vi "LC-MISDK_UserCalibration_sub.vi"(5 ".NET refnum入力":refnum<k24>, 6 "Color Space":T9(ring), 7 "Clust refnum":refnum<vi>) -> ()   [LabVIEW 2015]
uses:
  C:/Users/e09031/Documents/GMA/LC-160/Labview/Sample_LC-MISDK/LC-MISDK.dll
  LC-MISDK.dll
panel:
  in  "After_B":T1
  in  "After_G":T2
  in  "After_R":T3
  in  "After_W":T4
  in  "Before_B":T5
  in  "Before_G":T6
  in  "Before_R":T7
  in  "Before_W":T8
  out "Error Message":string
  in  "EXIT":bool
  in  "Calib":bool
  in  "ID":string
  out "Calib.Ch":T10(ring)
  out "Type of Calibration":enum32{"Single-Point", "RGB", "WRGB"}(radio)
  # "Value before Calibration"
  # "Value after Calibration"
  # "Lavel1"
  # "Lavel2"
  # "Lavel3"
  # "Lavel1"
  # "Lavel2"
  # "Lavel3"
  # "White"
  # "White"
  # "Red"
  # "Red"
  # "Green"
  # "Green"
  # "Blue"
  # "Blue"
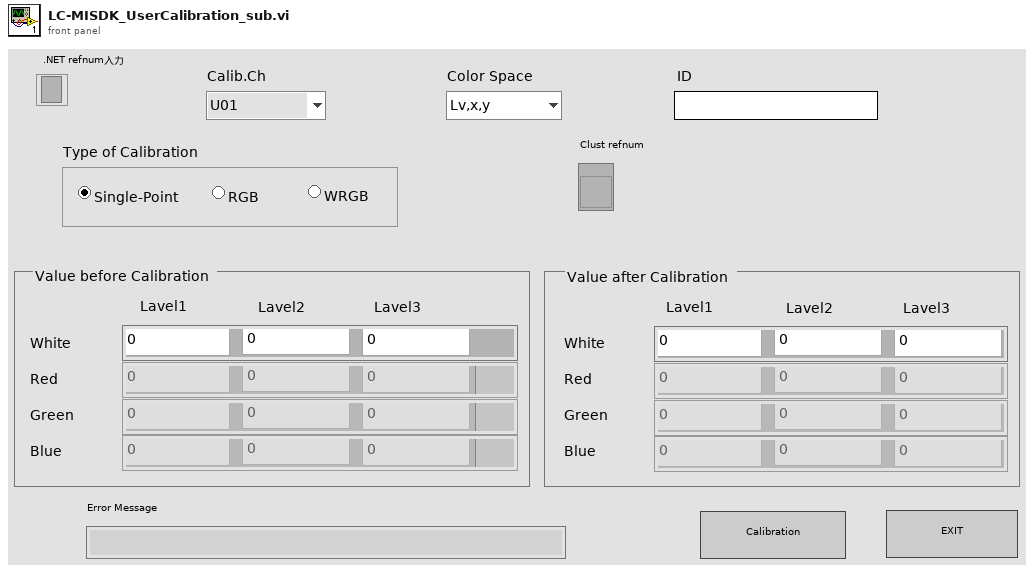
[diagram p1: front panel]
types:
  T1 = cluster{"After_B1":dbl, "After_B2":dbl, "After_B3":dbl}
  T2 = cluster{"After_G1":dbl, "After_G2":dbl, "After_G3":dbl}
  T3 = cluster{"After_R1":dbl, "After_R2":dbl, "After_R3":dbl}
  T4 = cluster{"After_W1":dbl, "After_W2":dbl, "After_W3":dbl}
  T5 = cluster{"before_B1":dbl, "Before_B":bool, "Before_B2":dbl, "Before_B3":dbl}
  T6 = cluster{"before_G1":dbl, "Before_G":bool, "Before_G2":dbl, "Before_G3":dbl}
  T7 = cluster{"before_R1":dbl, "Before_R":bool, "Before_R2":dbl, "Before_R3":dbl}
  T8 = cluster{"before_W1":dbl, "Before_W2":dbl, "Before_W3":dbl}
  T9 = enum16{"Lv,x,y", "Lv,u',v'", "Lv,Tcp,duv", "X,Y,Z", "Lv,λd,Pe"}
  T10 = enum16{"U01", "U02", "U03", "U04", "U05", "U06", "U07", "U08", "U09", "U10"}
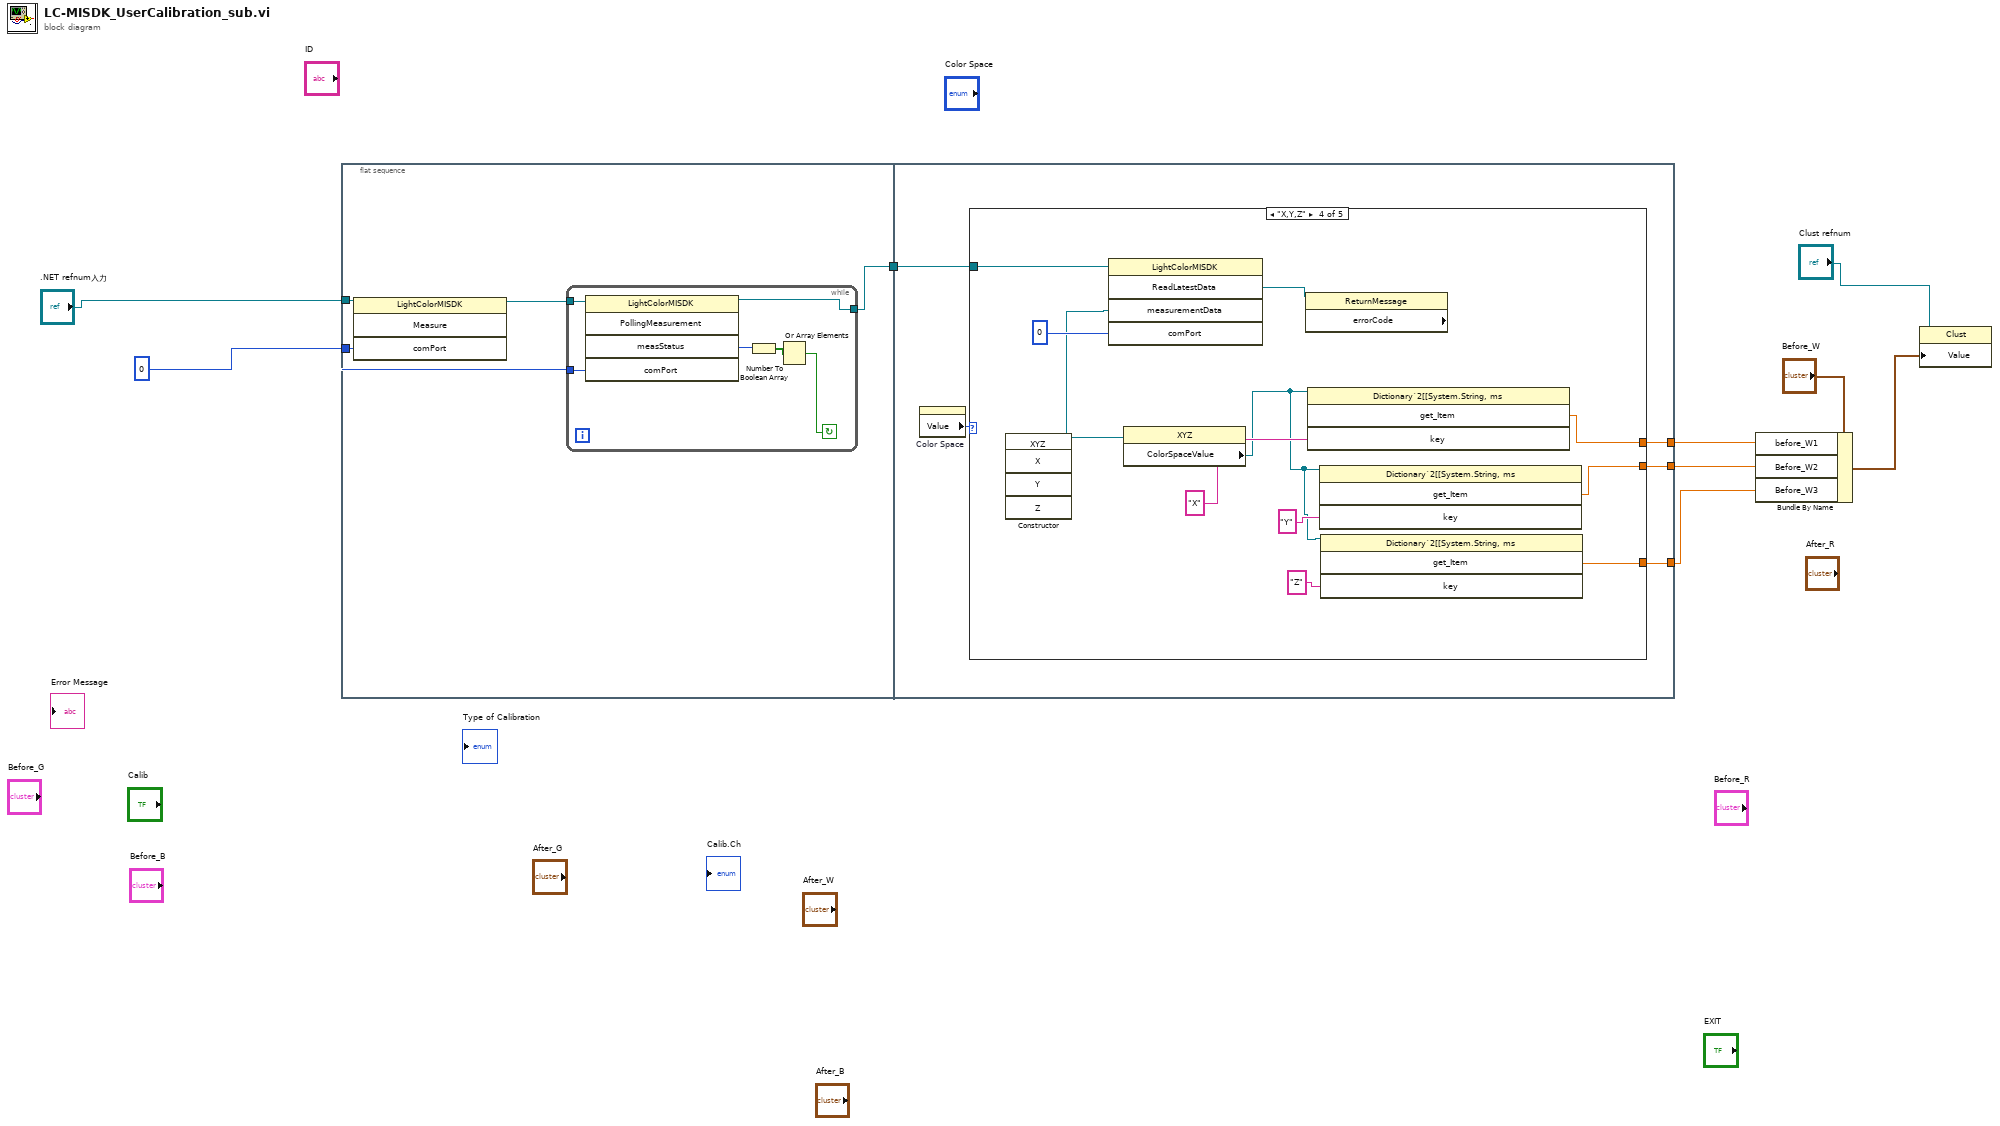
[diagram p0: block diagram]
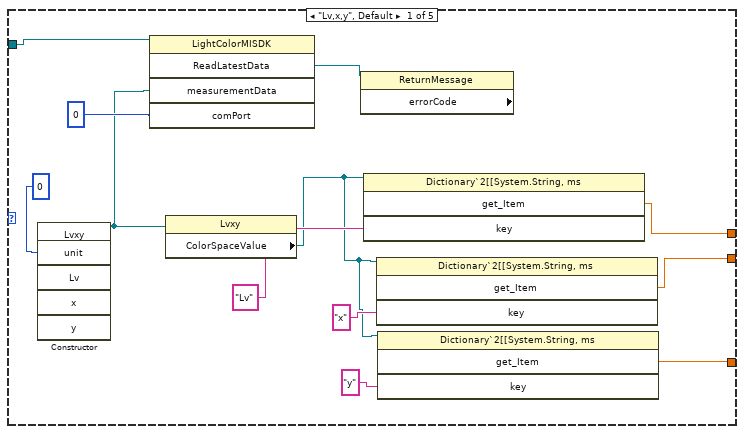
[diagram p2: hidden frame]
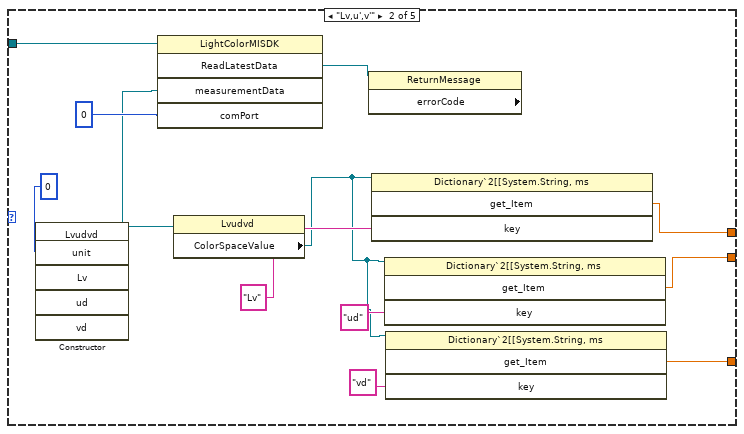
[diagram p3: hidden frame]
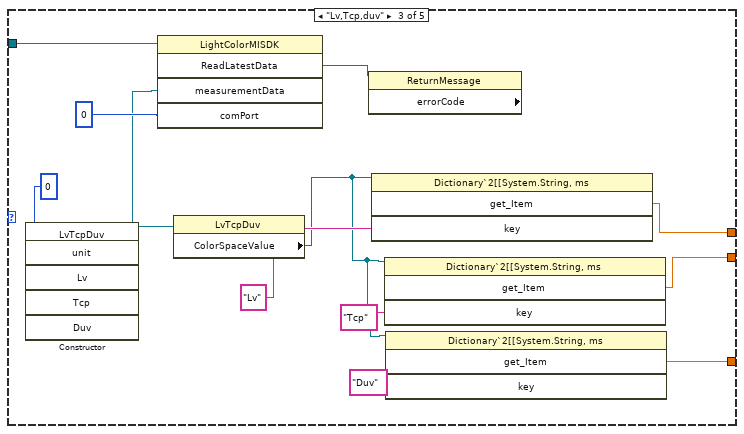
[diagram p4: hidden frame]
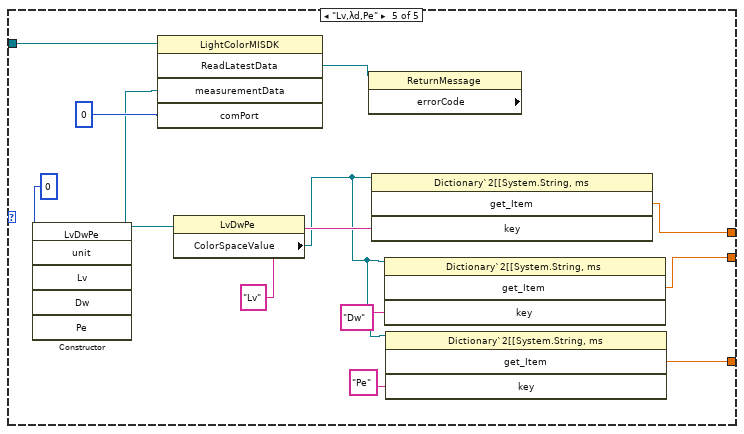
[diagram p5: hidden frame]
diagram:
  n1 = flat-sequence {
    tunnel: ".NET refnum入力" -> [w12]
    tunnel: 0 -> [w11]
    tunnel: [w10] -> w9
    tunnel: w9 -> [w24]
    tunnel: [w23] -> w8
    tunnel: [w22] -> w7
    tunnel: [w21] -> w6
    frame #0 {
      n2 = invoke on="インボークノード" class="LightColorMISDK" method="Measure"(reference=w12, "comPort"=w11) -> (reference out=w13:refnum<k24>)  [unwired: 2 in, 3 out]
      n3 = while {
        tunnel: [w18] -> w10
        tunnel: w13 -> [w17]
        tunnel: w11 -> [w14]
        stop <- w15 continue-if-true
        n4 = invoke on="インボークノード" class="LightColorMISDK" method="PollingMeasurement"(reference=w17, "comPort"=w14) -> (reference out=w18:refnum<k24>, "measStatus"=w19:i32)  [unwired: 3 in, 3 out]
        n5 = Number To Boolean Array(number=w19) -> (Boolean array=w16:bool[])
        n6 = Or Array Elements(Boolean array=w16) -> (logical OR=w15:bool)
      }
    }
    frame #1 {
      n7 = property on="Color Space" class="Enum （指定）"() -> ("Value"=w20:T9)  [unwired: 2 in, 2 out]
      n8 = case shown="\"X,Y,Z\"" w20 {
        tunnel: w24 -> [w28 w40 w52 w64 w75]
        tunnel: [w27 w39 w51 w63 w74] -> w23
        tunnel: [w26 w38 w50 w62 w73] -> w22
        tunnel: [w25 w37 w49 w61 w72] -> w21
        frame "Lv,x,y", Default {
          n9 = constructor class="Lvxy"("unit"=0) -> (reference out=w34:refnum<k24>)  [unwired: 6 in, 6 out]
          n10 = invoke on="インボークノード" class="LightColorMISDK" method="ReadLatestData"(reference=w28, "measurementData"=w34, "comPort"=0) -> ("ReadLatestData"=w35:refnum<k24>)  [unwired: 2 in, 4 out]
          n11 = property class="Lvxy"(reference=w34) -> ("ColorSpaceValue"=w31:refnum<k24>)  [unwired: 1 in, 2 out]
          n12 = property on="プロパティノード" class="ReturnMessage" props=["errorCode"](reference=w35) -> ()  [unwired: 1 in, 3 out]
          n13 = invoke class="Dictionary`2[[System.String, ms" method="get_Item"(reference=w31, "key"="Lv") -> ("get_Item"=w27:dbl)  [unwired: 2 in, 3 out]
          n14 = invoke class="Dictionary`2[[System.String, ms" method="get_Item"(reference=w31, "key"="x") -> ("get_Item"=w26:dbl)  [unwired: 2 in, 3 out]
          n15 = invoke class="Dictionary`2[[System.String, ms" method="get_Item"(reference=w31, "key"="y") -> ("get_Item"=w25:dbl)  [unwired: 2 in, 3 out]
        }
        frame "Lv,u',v'" {
          n16 = constructor class="Lvudvd"("unit"=0) -> (reference out=w46:refnum<k24>)  [unwired: 6 in, 6 out]
          n17 = invoke on="インボークノード" class="LightColorMISDK" method="ReadLatestData"(reference=w40, "measurementData"=w46, "comPort"=0) -> ("ReadLatestData"=w47:refnum<k24>)  [unwired: 2 in, 4 out]
          n18 = property class="Lvudvd"(reference=w46) -> ("ColorSpaceValue"=w43:refnum<k24>)  [unwired: 1 in, 2 out]
          n19 = property on="プロパティノード" class="ReturnMessage" props=["errorCode"](reference=w47) -> ()  [unwired: 1 in, 3 out]
          n20 = invoke class="Dictionary`2[[System.String, ms" method="get_Item"(reference=w43, "key"="Lv") -> ("get_Item"=w39:dbl)  [unwired: 2 in, 3 out]
          n21 = invoke class="Dictionary`2[[System.String, ms" method="get_Item"(reference=w43, "key"="ud") -> ("get_Item"=w38:dbl)  [unwired: 2 in, 3 out]
          n22 = invoke class="Dictionary`2[[System.String, ms" method="get_Item"(reference=w43, "key"="vd") -> ("get_Item"=w37:dbl)  [unwired: 2 in, 3 out]
        }
        frame "Lv,Tcp,duv" {
          n23 = constructor class="LvTcpDuv"("unit"=0) -> (reference out=w58:refnum<k24>)  [unwired: 6 in, 6 out]
          n24 = invoke on="インボークノード" class="LightColorMISDK" method="ReadLatestData"(reference=w52, "measurementData"=w58, "comPort"=0) -> ("ReadLatestData"=w59:refnum<k24>)  [unwired: 2 in, 4 out]
          n25 = property class="LvTcpDuv"(reference=w58) -> ("ColorSpaceValue"=w55:refnum<k24>)  [unwired: 1 in, 2 out]
          n26 = property on="プロパティノード" class="ReturnMessage" props=["errorCode"](reference=w59) -> ()  [unwired: 1 in, 3 out]
          n27 = invoke class="Dictionary`2[[System.String, ms" method="get_Item"(reference=w55, "key"="Lv") -> ("get_Item"=w51:dbl)  [unwired: 2 in, 3 out]
          n28 = invoke class="Dictionary`2[[System.String, ms" method="get_Item"(reference=w55, "key"="Tcp") -> ("get_Item"=w50:dbl)  [unwired: 2 in, 3 out]
          n29 = invoke class="Dictionary`2[[System.String, ms" method="get_Item"(reference=w55, "key"="Duv") -> ("get_Item"=w49:dbl)  [unwired: 2 in, 3 out]
        }
        frame "X,Y,Z" {
          n30 = constructor class="XYZ"() -> (reference out=w69:refnum<k24>)  [unwired: 6 in, 5 out]
          n31 = invoke on="インボークノード" class="LightColorMISDK" method="ReadLatestData"(reference=w64, "measurementData"=w69, "comPort"=0) -> ("ReadLatestData"=w70:refnum<k24>)  [unwired: 2 in, 4 out]
          n32 = property class="XYZ"(reference=w69) -> ("ColorSpaceValue"=w66:refnum<k24>)  [unwired: 1 in, 2 out]
          n33 = property on="プロパティノード" class="ReturnMessage" props=["errorCode"](reference=w70) -> ()  [unwired: 1 in, 3 out]
          n34 = invoke class="Dictionary`2[[System.String, ms" method="get_Item"(reference=w66, "key"="X") -> ("get_Item"=w63:dbl)  [unwired: 2 in, 3 out]
          n35 = invoke class="Dictionary`2[[System.String, ms" method="get_Item"(reference=w66, "key"="Y") -> ("get_Item"=w62:dbl)  [unwired: 2 in, 3 out]
          n36 = invoke class="Dictionary`2[[System.String, ms" method="get_Item"(reference=w66, "key"="Z") -> ("get_Item"=w61:dbl)  [unwired: 2 in, 3 out]
        }
        frame "Lv,λd,Pe" {
          n37 = constructor class="LvDwPe"("unit"=0) -> (reference out=w81:refnum<k24>)  [unwired: 6 in, 6 out]
          n38 = invoke on="インボークノード" class="LightColorMISDK" method="ReadLatestData"(reference=w75, "measurementData"=w81, "comPort"=0) -> ("ReadLatestData"=w82:refnum<k24>)  [unwired: 2 in, 4 out]
          n39 = property class="LvDwPe"(reference=w81) -> ("ColorSpaceValue"=w78:refnum<k24>)  [unwired: 1 in, 2 out]
          n40 = property on="プロパティノード" class="ReturnMessage" props=["errorCode"](reference=w82) -> ()  [unwired: 1 in, 3 out]
          n41 = invoke class="Dictionary`2[[System.String, ms" method="get_Item"(reference=w78, "key"="Lv") -> ("get_Item"=w74:dbl)  [unwired: 2 in, 3 out]
          n42 = invoke class="Dictionary`2[[System.String, ms" method="get_Item"(reference=w78, "key"="Dw") -> ("get_Item"=w73:dbl)  [unwired: 2 in, 3 out]
          n43 = invoke class="Dictionary`2[[System.String, ms" method="get_Item"(reference=w78, "key"="Pe") -> ("get_Item"=w72:dbl)  [unwired: 2 in, 3 out]
        }
      }
    }
  }
  n44 = Bundle By Name(cluster="Before_W", "before_W1"=w8, "Before_W2"=w7, "Before_W3"=w6) -> (w3:T8)
  n45 = property class="Clust"(reference="Clust refnum", "Value"=w3) -> ()  [unwired: 1 in, 2 out]
